vi "Draw Expanded Terminals.vi"(6 "State":T7, 7 "Sizes":T6, 9 "Expanded Types":T1[](array[typedef]), 11 "Picture  In":picture) -> (3 "Picture":picture)   [LabVIEW 2020, in "FlexBlock.xnode"]
uses:
  FlexBlock.xnode
  State.ctl
  FlexBlocks/Type Descriptor.ctl
  FlexBlocks/Terminal Direction.ctl
  FlexBlocks/Value Mode.ctl
  FlexBlocks/Terminal State.ctl
  FlexBlocks/Special Terminal.ctl
  FlexBlocks/Errors.ctl
  <vilib>/picture/picture.llb/imagedata.ctl
  FlexBlocks/Calculated Sizes.ctl
  FlexBlocks/Size Constants.ctl
  FlexBlocks/FlexBlocks.lvlib
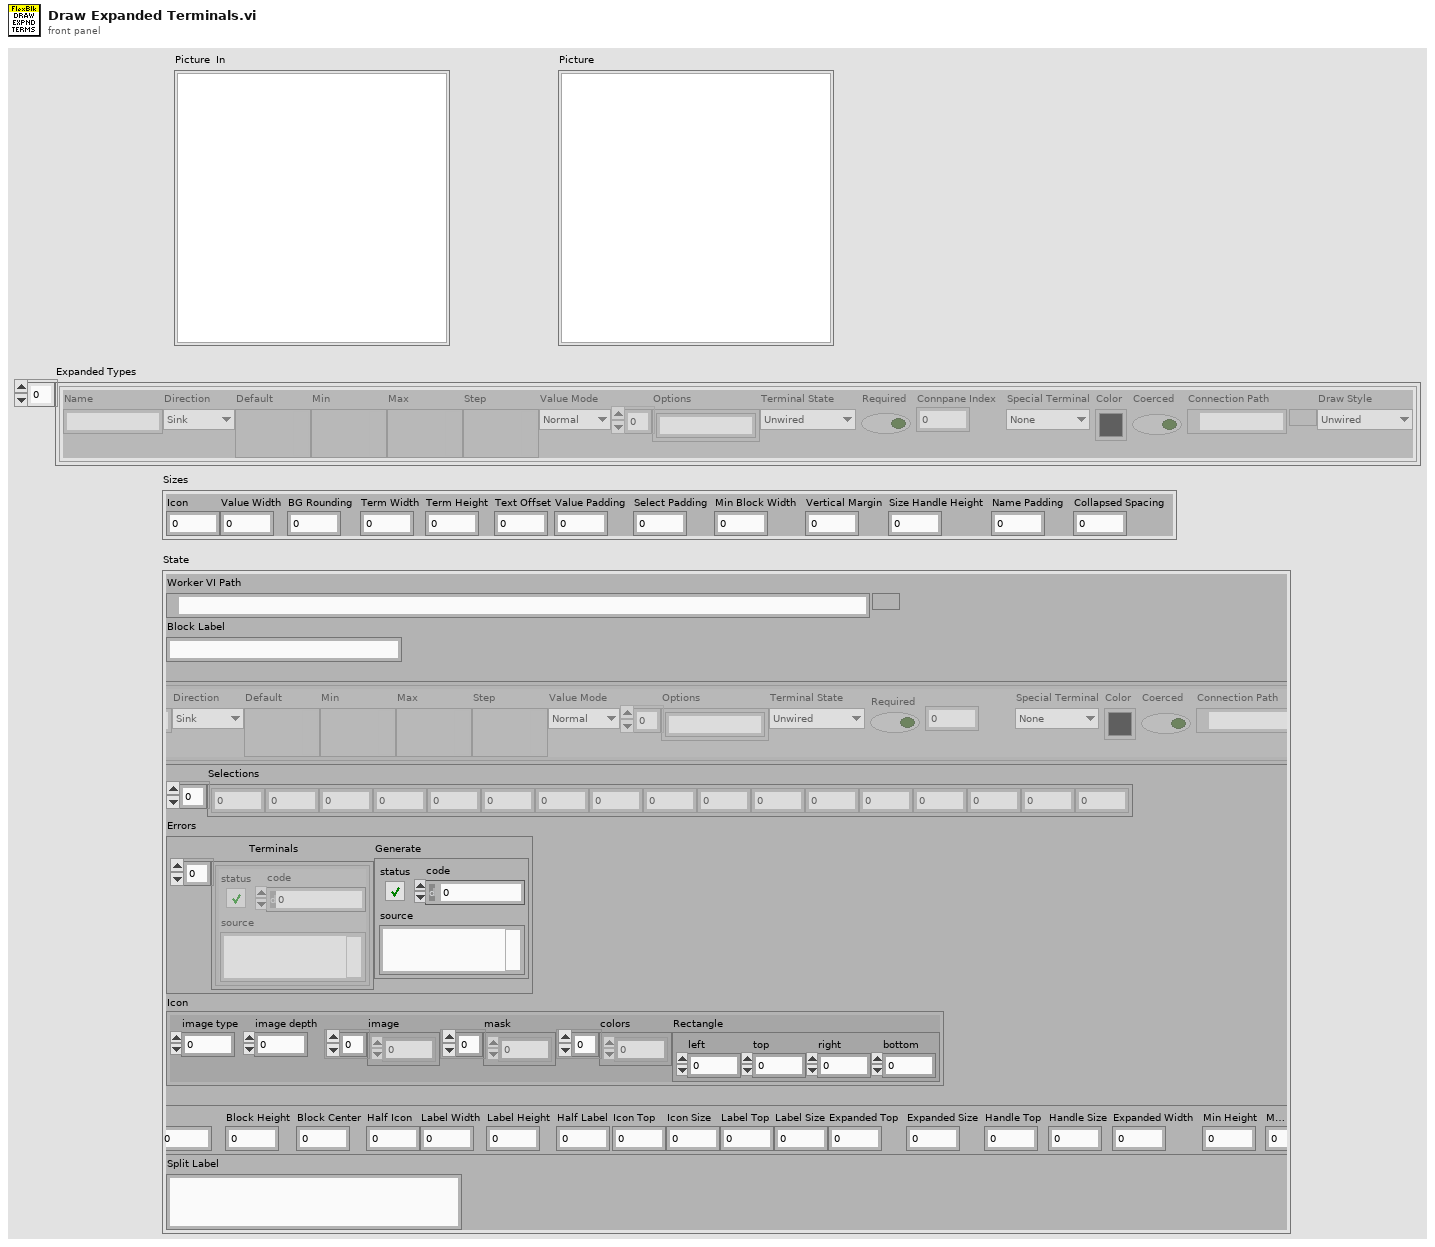
[diagram p1: front panel]
types:
  T1 = typedef "FlexBlocks.lvlib/Type Descriptor.ctl" = cluster{"Name":string, "Direction":T2, "Default":variant, "Min":variant, "Max":variant, "Step":variant, "Value Mode":T3, "Options":string[], "Terminal State":T4, "Required":bool, "Connpane Index":i32, "Special Terminal":T5, "Color":u32, "Coerced":bool, "Connection Path":path, "Draw Style":T4}
  T2 = typedef "FlexBlocks.lvlib/Terminal Direction.ctl" = enum16{"Sink", "Source"}
  T3 = typedef "FlexBlocks.lvlib/Value Mode.ctl" = enum16{"Normal", "Range", "Select"}
  T4 = typedef "FlexBlocks.lvlib/Terminal State.ctl" = enum16{"Unwired", "BadType", "BadRef", "Channel", "Value", "Control Ref"}
  T5 = typedef "FlexBlocks.lvlib/Special Terminal.ctl" = enum16{"None", "Action", "Init", "Tag", "State in", "State out", "Error"}
  T6 = typedef "FlexBlocks.lvlib/Size Constants.ctl" = cluster{"Icon":i32, "Value Width":i32, "BG Rounding":i32, "Term Width":i32, "Term Height":i32, "Text Offset":i32, "Value Padding":i32, "Select Padding":i32, "Min Block Width":i32, "Vertical Margin":i32, "Size Handle Height":i32, "Name Padding":i32, "Collapsed Spacing":i32}
  T7 = typedef "FlexBlock.xnode/State.ctl" = cluster{"Worker VI Path":path, "Block Label":string, "Types":T1[], "Selections":i32[], "Errors":T8, "Icon":T9, "Calcd Sizes":T10, "Split Label":string}
  T8 = typedef "FlexBlocks.lvlib/Errors.ctl" = cluster{"Terminals":errorcluster[], "Generate":errorcluster}
  T9 = typedef "imagedata.ctl" = cluster{"image type":i32, "image depth":i32, "image":u8[], "mask":u8[], "colors":u32[], "Rectangle":cluster{"left":i16, "top":i16, "right":i16, "bottom":i16}}
  T10 = typedef "FlexBlocks.lvlib/Calculated Sizes.ctl" = cluster{"Text Width":i32, "Text Height":i32, "Half Text":i32, "Block Width":i32, "Block Height":i32, "Block Center":i32, "Half Icon":i32, "Label Width":i32, "Label Height":i32, "Half Label":i32, "Icon Top":i32, "Icon Size":i32, "Label Top":i32, "Label Size":i32, "Expanded Top":i32, "Expanded Size":i32, "Handle Top":i32, "Handle Size":i32, "Expanded Width":i32, "Min Height":i32, "Max Height":i32}
  T11 = cluster{"left":i16, "top":i16, "right":i16, "bottom":i16}
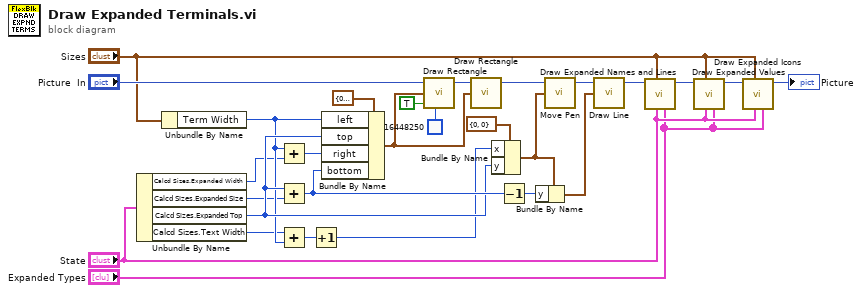
[diagram p0: block diagram]
diagram:
  n1 = Unbundle By Name("State") -> ("Calcd Sizes.Expanded Width"=w8:i32, "Calcd Sizes.Expanded Size"=w9:i32, "Calcd Sizes.Expanded Top"=w17:i32, "Calcd Sizes.Text Width"=w7:i32)
  n2 = Unbundle By Name("Sizes") -> ("Term Width"=w16:i32)
  n3 = Add(x=w16, y=w8) -> (x+y=w24:i32)
  n4 = Add(x=w17, y=w9) -> (x+y=w19:i32)
  n5 = Add(x=w7, y=w16) -> (x+y=w15:i32)
  n6 = Increment(x=w15) -> (x+1=w6:i32)
  n7 = Bundle By Name(cluster=T11 {"left"=0, "top"=0, "right"=0, "bottom"=0} ("rect"), "left"=w16, "top"=w17, "right"=w24, "bottom"=w19) -> (w22:T11)
  n8 = call <vilib>:"Draw Rectangle.vi"("picture"="Picture  In", "rect"=w22, "fill?(F)"=TRUE, "color(black)"=u32 16448250) -> ("new picture"=w23:picture)  [unwired: 5 in]
  n9 = call <vilib>:"Draw Rectangle.vi"("picture"=w23, "rect"=w22) -> ("new picture"=w21:picture)  [unwired: 7 in]
  n10 = Bundle By Name(cluster=cluster{"x":i16, "y":i16} {"x"=0, "y"=0} ("new position"), "x"=w6, "y"=w17) -> (w18:cluster{"x":i16, "y":i16})
  n11 = Decrement(x=w19) -> (x-1=w12:i32)
  n12 = Bundle By Name(cluster=w18, "y"=w12) -> (w14:cluster{"x":i16, "y":i16})
  n13 = call <vilib>:"Move Pen.vi"("new position"=w18, "picture"=w21) -> ("new picture"=w13:picture)  [unwired: 3 in]
  n14 = call <vilib>:"Draw Line.vi"("picture"=w13, "end point"=w14) -> ("new picture"=w11:picture)  [unwired: 7 in]
  n15 = call "Draw Expanded Names and Lines.vi"("Expanded Types"="Expanded Types", "State"="State", "Sizes"="Sizes", "Picture  In"=w11) -> ("Picture"=w10:picture)  [unwired: 7 in]
  n16 = call "Draw Expanded Values.vi"("Expanded Types"="Expanded Types", "State"="State", "Sizes"="Sizes", "Picture  In"=w10) -> ("Picture"=w5:picture)  [unwired: 7 in]
  n17 = call "Draw Expanded Icons.vi"("Expanded Types"="Expanded Types", "State"="State", "Sizes"="Sizes", "Picture  In"=w5) -> ("Picture"=→"Picture":picture)  [unwired: 7 in]
